vi "Microscope.SetDependencies.vi"(8 "error in (no error)":errorcluster, 10 "Dependencies":T1, 11 "Microscope":refnum<class "Microscope.lvclass">) -> (0 "error out":errorcluster, 3 "Microscope out":refnum<class "Microscope.lvclass">)   [LabVIEW 2013, in "Microscope.lvclass"]
doc: "---------------------------------------------------------------\nJKI State Machine Objects™\nhttp://jki.net/state-machine-objects/\nCopyright (C) 2005-2015, JKI <info@jki.net>\nALL RIGHTS RESERVEDJKI State Machine Objects (SMO) 1.0.0.5\nJKI - JKI\nCopyright (c) 2016, JKI"
uses:
  Microscope.lvclass
  XYStage/XYStage.lvclass
  Camera/Camera.lvclass
  Typedefs/Dependencies--Cluster.ctl
panel:
  # "For instructions on how to use the JKI State Machine Objects, examples and video tutorials, visit:\nhttp://jki.net/state-machine-objects/\n\nJKI State Machine Objects™\nhttp://jki.net/state-machine-objects/\nCopyright (C) 2005-2015, JKI <info@jki.net>\nALL RIGHTS RESERVED"
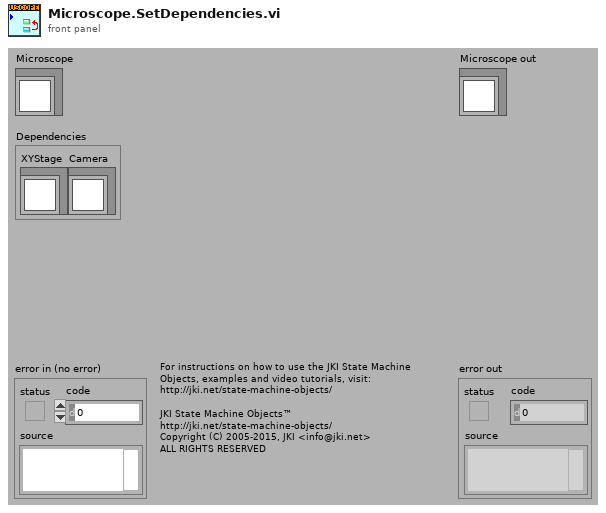
[diagram p1: front panel]
types:
  T1 = typedef "Microscope.lvclass/Dependencies--Cluster.ctl" = cluster{"XYStage":refnum<class "XYStage.lvclass">, "Camera":refnum<class "Camera.lvclass">}
  T2 = typedef "Microscope.lvclass/PrivateData--Ref.ctl" = refnum<data-value>
  T3 = typedef "Microscope.lvclass/PrivateData--Cluster.ctl" = cluster{"Public Events":T4, "Protected Events":T5, "Private Events":T6, "Dependencies":T1, "Configuration":T7}
  T4 = typedef "Microscope.lvclass/PublicEvents--Cluster.ctl" = cluster{"Value Changed":refnum<user-event>, "Initialized":refnum<user-event>}
  T5 = typedef "Microscope.lvclass/ProtectedEvents--Cluster.ctl" = cluster{"placeholder":refnum<user-event>}
  T6 = typedef "Microscope.lvclass/PrivateEvents--Cluster.ctl" = cluster{"New Value":refnum<user-event>, "Initialize":refnum<user-event>, "CaptureImageAtPosition":refnum<user-event>}
  T7 = typedef "Microscope.lvclass/Configuration--Cluster.ctl" = cluster{"XY Stage":string, "Camera":string, "image output folder":path, "filetype":string}
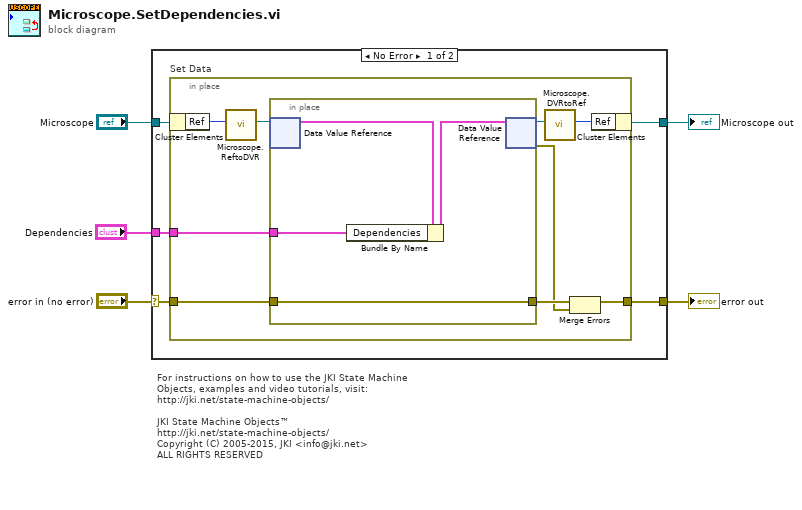
[diagram p0: block diagram]
diagram:
  # "For instructions on how to use the JKI State Machine Objects, examples and video tutorials, visit:\nhttp://jki.net/state-machine-objects/\n\nJKI State Machine Objects™\nhttp://jki.net/state-machine-objects/\nCopyright (C) 2005-2015, JKI <info@jki.net>\nALL RIGHTS RESERVED"
  n1 = case shown="No Error" "error in (no error)" {
    selector: "error in (no error)" -> [w8 w24]
    tunnel: "Microscope" -> [w9 w25]
    tunnel: [w6 w24] -> w4
    tunnel: [w7 w25] -> w3
    tunnel: "Dependencies" -> [w10 _]
    frame No Error {
      n2 = in-place "Set Data" {
        in-place-border: w8 -> [w19]
        in-place-border: [w17] -> w6
        in-place-border: w10 -> [w16]
        n3 = in-place-cluster #1(w9) -> ("Ref"=w15:u32)
        n4 = call "Microscope.ReftoDVR.vi"("Ref"=w15) -> ("Ref"=w14:T2)  [unwired: 10 in]
        n5 = in-place {
          in-place-border: w19 -> [w23]
          in-place-border: [w23] -> w18
          in-place-border: w16 -> [w20]
          n6 = in-place-dvr #2(w14) -> (w21:T3)  [unwired: 1 out]
          n7 = Bundle By Name(cluster=w21, "Dependencies"=w20) -> (w22:T3)
          n8 = in-place-dvr #2(w22) -> (w13:T2, w11:errorcluster)
        }
        n9 = call "Microscope.DVRtoRef.vi"("Ref"=w13) -> ("Ref"=w12:u32)  [unwired: 10 in]
        n10 = Merge Errors(w18, w11) -> (w17:errorcluster)
        n11 = in-place-cluster #1("Ref"=w12) -> (w7:refnum<class "Microscope.lvclass">)
      }
    }
    frame Error {
    }
  }
  "error out" <- w4
  "Microscope out" <- w3
